vi "Load.vi"(0 "iUser Configuration Manager DVR":refnum<data-value>, 5 "Username":string, 7 "Password":string, 9 "Path":path, 11 "error in":errorcluster, 12 "Persistence":refnum<class "IPersist.lvclass">) -> (4 "dup iUser Configuration Manager DVR":refnum<data-value>, 6 "Verified":bool, 8 "Verification Message":string, 15 "error out":errorcluster)   [LabVIEW 2019, in "User Configuration Manager.lvlib" / "By Ref.lvlib"]
doc: "Loads the User Configuration Manager from disk and logs in using the credentials specified. A user with the credentials specified must exist in the User Configuration Manager."
uses:
  <vilib>/gpm_packages/@cs/user-manager/Source/User Configuration Manager Ref/By Ref.lvlib
  <vilib>/gpm_packages/@cs/user-manager/Source/iUser Configuration Manager/iUser Configuration Manager.lvclass
  <vilib>/gpm_packages/@cs/persistence/source/IPersist/IPersist.lvclass
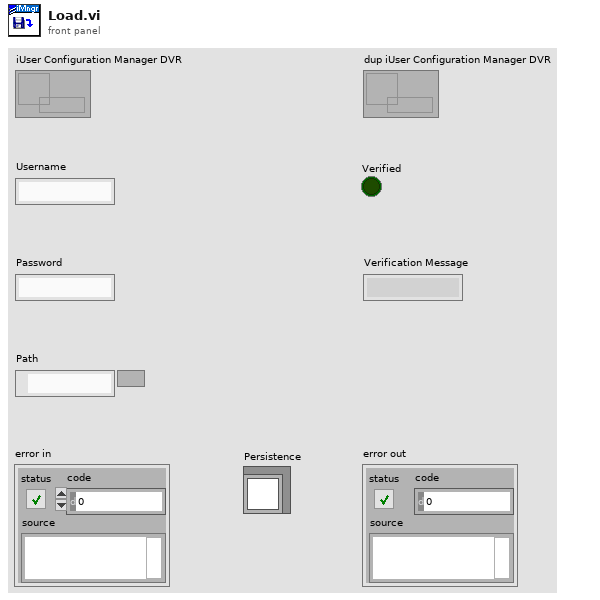
[diagram p1: front panel]
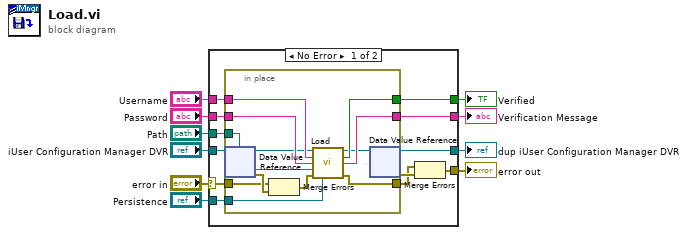
[diagram p0: block diagram]
diagram:
  n1 = case shown="No Error" "error in" {
    selector: "error in" -> [w20 w36]
    tunnel: "iUser Configuration Manager DVR" -> [w22 w35]
    tunnel: [w21 w36] -> w9
    tunnel: [w17 w35] -> w7
    tunnel: "Username" -> [w16 _]
    tunnel: "Password" -> [w15 _]
    tunnel: "Path" -> [w14 _]
    tunnel: "Persistence" -> [w13 _]
    tunnel: [w12 _] -> w2
    tunnel: [w11 _] -> w1
    frame No Error {
      n2 = in-place "IPES" {
        in-place-border: [w30] -> w18
        in-place-border: w20 -> [w33]
        in-place-border: w16 -> [w29]
        in-place-border: w15 -> [w25]
        in-place-border: w14 -> [w28]
        in-place-border: w13 -> [w26]
        in-place-border: [w32] -> w12
        in-place-border: [w31] -> w11
        n3 = in-place-dvr #1(w22) -> (w24:refnum<class "iUser Configuration Manager.lvclass">, w34:errorcluster)
        n4 = Merge Errors(w33, w34) -> (w27:errorcluster)
        n5 = call-dynamic "Load.vi"("iUser Configuration Manager"=w24, "Username"=w29, "Password"=w25, "Path"=w28, "error in (no error)"=w27, "Persistence"=w26) -> ("iUser Configuration Manager.lvclass"=w23:refnum<class "iUser Configuration Manager.lvclass">, "Verified"=w32:bool, "Verification Message"=w31:string, "error out"=w30:errorcluster)  [unwired: 6 in]
        n6 = in-place-dvr #1(w23) -> (w17:refnum<data-value>, w19:errorcluster)
      }
      n7 = Merge Errors(w18, w19) -> (w21:errorcluster)
    }
    frame Error {
    }
  }
  "error out" <- w9
  "dup iUser Configuration Manager DVR" <- w7
  "Verified" <- w2
  "Verification Message" <- w1
